vi "InsertDataIntoQueue_ProjectBase.vi"(8 "error in (no error)":errorcluster, 9 "RxData":string, 10 "Consumer State":T1, 11 "Queue in":refnum<queue>) -> (0 "error out":errorcluster, 3 "queue out":refnum<queue>)   [LabVIEW 2019]
uses:
  QueueCluster_ProjectBase.ctl
  ConsumerStates_ProjectBase.ctl
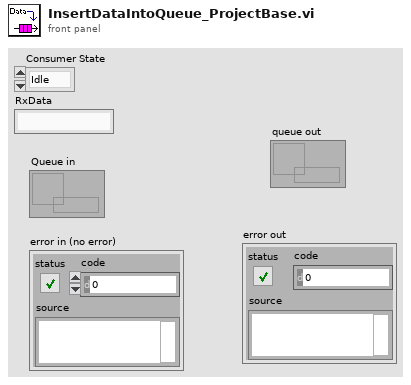
[diagram p1: front panel]
types:
  T1 = typedef "ConsumerStates_ProjectBase.ctl" = enum16{"Idle", "Generate TDMS", "Heating Sensor", "Catch Data", "Error"}
  T2 = typedef "QueueCluster_ProjectBase.ctl" = cluster{"error constant":errorcluster, "Consumer State":T1, "RxData":string}
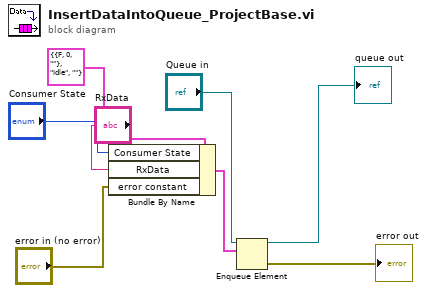
[diagram p0: block diagram]
diagram:
  n1 = Bundle By Name(cluster=T2 {"error constant"={"status"=FALSE, "code"=0, "source"=""}, "Consumer State"=enum."Idle", "RxData"=""}, "Consumer State"="Consumer State", "RxData"="RxData", "error constant"="error in (no error)") -> (w6:T2)
  n2 = Enqueue Element(queue="Queue in", element=w6) -> (queue out=→"queue out":refnum<queue>, error out=→"error out":errorcluster)  [unwired: 2 in, 1 out]
